vi "PromVIEW Instantiate WS Dialog.vi"(11 "Project Refnum":refnum<vi>) -> (1 "Cancelled":bool, 2 "Web Resources Base Path out":path, 3 "Web Service Name out":string)   [LabVIEW 2020]
panel:
  in  "Web Resources Base Path":path
  in  "Web Service Name":string
  in  "Cancel":bool
  in  "Validate":bool
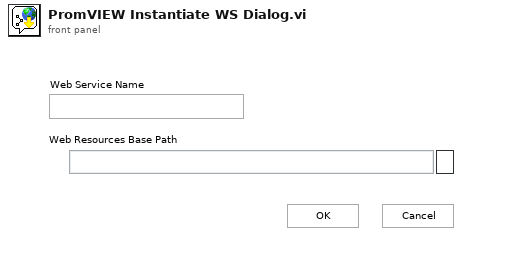
[diagram p1: front panel]
types:
  T1 = enum32{"Invalid", "Standard", "Closed", "Hidden", "Minimized", "Maximized"}
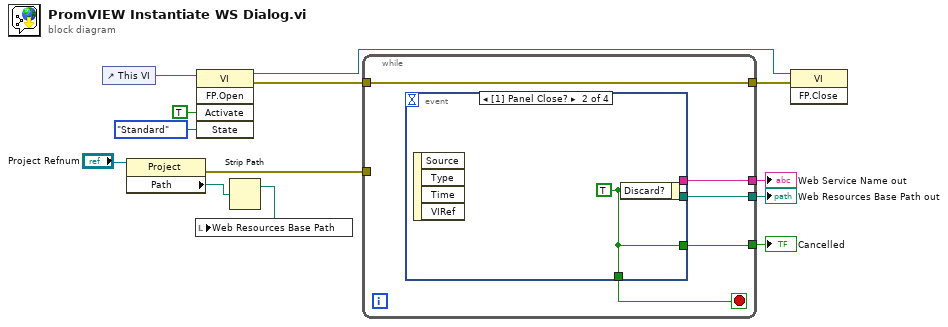
[diagram p0: block diagram]
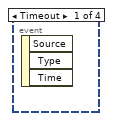
[diagram p2: hidden frame]
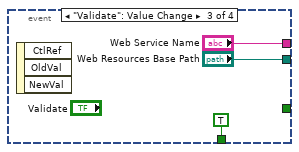
[diagram p3: hidden frame]
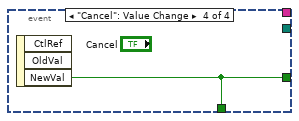
[diagram p4: hidden frame]
diagram:
  n1 = control-ref of="This VI"() -> (w6:refnum<vi>)
  n2 = property class="Project"(reference="Project Refnum") -> (error out=w7:errorcluster, "Path"=w9:path)  [unwired: 1 in, 1 out]
  n3 = invoke class="VI" method="FP.Open"(reference=w6, "Activate"=TRUE ("Activate?"), "State"=T1."Standard") -> (reference out=w2:refnum<vi>, error out=w3:errorcluster)  [unwired: 2 in, 3 out]
  n4 = Strip Path(path=w9) -> (stripped path=w8:path)  [unwired: 1 out]
  n5 = local write "Web Resources Base Path"(w8) -> ()
  n6 = while {
    tunnel: [w17] -> w13
    tunnel: [w16] -> w12
    tunnel: [w15] -> w11
    tunnel: w7 -> [_]
    tunnel: w3 -> [w14]
    tunnel: [w14] -> w1
    stop <- w18 stop-if-true
    n7 = event shown="[1] Panel Close?" {
      selector: _ -> [_ _ _ _]
      dyn-events: _ -> [_ _ _ _]
      timeout: _ -> [_ _ _ _]
      tunnel: [_ w19 TRUE ("Discard?") w23] -> w18
      tunnel: [_ w19 _ w23] -> w17
      tunnel: [_ _ "Web Service Name" _] -> w16
      tunnel: [_ _ "Web Resources Base Path" _] -> w15
      event Timeout {
        n8 = event-data() -> ()  [unwired: 1 in, 3 out]
      }
      event Panel Close? {
        w19 = TRUE ("Discard?")
        n9 = event-data() -> ()  [unwired: 1 in, 4 out]
        n10 = event-data("Discard?"=w19) -> ()  [unwired: 1 in, 1 out]
      }
      event "Validate": Value Change {
        n11 = event-data() -> ()  [unwired: 1 in, 3 out]
      }
      event "Cancel": Value Change {
        n12 = event-data() -> ("NewVal"=w23:bool)  [unwired: 1 in, 2 out]
      }
    }
  }
  "Cancelled" <- w13
  "Web Service Name out" <- w12
  "Web Resources Base Path out" <- w11
  n13 = invoke class="VI" method="FP.Close"(reference=w2, error in=w1) -> ()  [unwired: 1 in, 3 out]
